vi "Loading.vi"(3 "error in":errorcluster caption="error in (no error)", 4 "reference":refnum<vi>, 5 "Value":u8) -> (0 "error out":errorcluster)   [LabVIEW 2017]
doc: "Displays a standard dialog box that prompts users to enter information, such as a user name and password.\n--------------------\n\nThis Express VI is configured as follows:\n\nMessage to Display to the User:\nThe inputs are: \nNumber: c002"
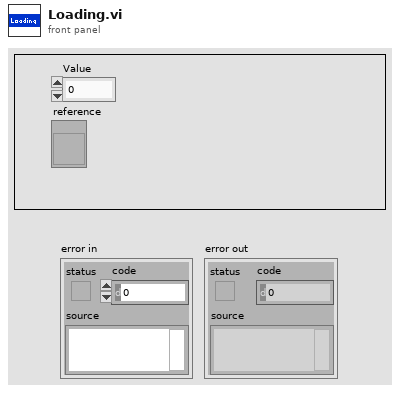
[diagram p1: front panel]
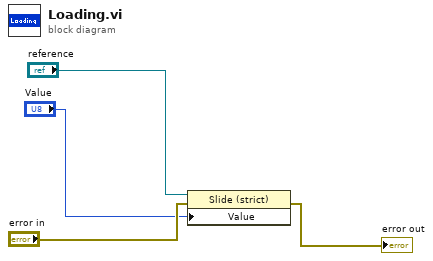
[diagram p0: block diagram]
diagram:
  n1 = property on="Property Node" class="Slide (strict)"(reference="reference", error in="error in", "Value"="Value") -> (error out=→"error out":errorcluster)  [unwired: 1 out]
